vi "Get configuration chain.vi"(8 "error in (no error)":errorcluster, 11 "ServiceManager in":refnum<class "ServiceManager.lvclass">) -> (0 "error out":errorcluster, 1 "class name":string[](array[string]), 2 "configuration chain":variant[](array[variant]), 3 "ServiceManager out":refnum<class "ServiceManager.lvclass">)   [LabVIEW 2012, in "ServiceManager.lvclass"]
doc: "Returns an array of variants containing the configuration clusters of each class in the inheritance chain (lowest child class first), together with an array of all class names in the inheritance chain.\n\nFor classes without configuration cluster, the configuration chain contains empty variants."
uses:
  ServiceManager.lvclass
  Murmex/LabVIEW/Murmex/Murmex/Murmex.lvclass
  ServiceManager.lvclass/ServiceManager.ctl
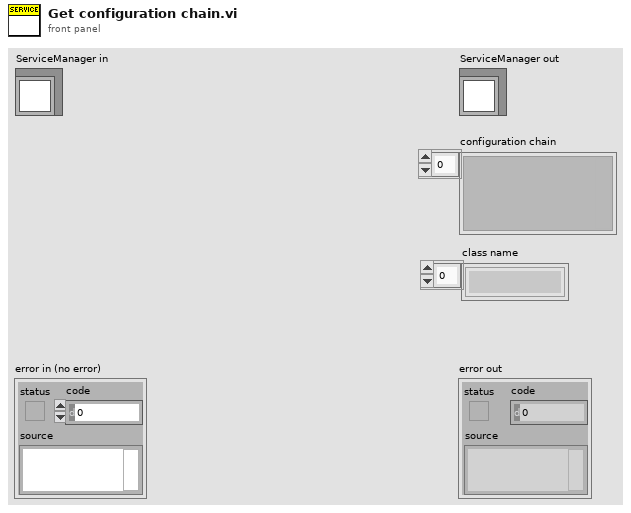
[diagram p1: front panel]
types:
  T1 = typedef "ServiceManager.lvclass/configuration_cluster.ctl" = cluster{"search paths":string[]}
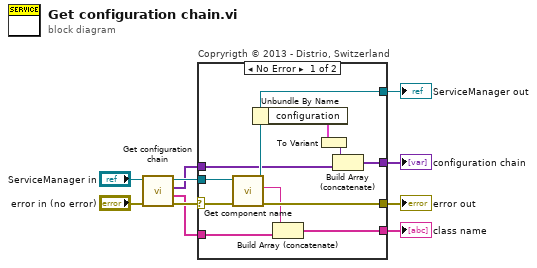
[diagram p0: block diagram]
diagram:
  n1 = call-parent "Get configuration chain.vi"("error in (no error)"="error in (no error)", "MurmexBase in"="ServiceManager in") -> ("error out"=w8:errorcluster, "class name"=w4:string[], "configuration chain"=w5:variant[], "MurmexBase out"=w7:refnum<class "ServiceManager.lvclass">)  [unwired: 6 in]
  n2 = case "Copryrigth © 2013 - Distrio, Switzerland" shown="No Error" w8 {
    selector: w8 -> [w18 w23]
    tunnel: [w17 w23] -> w1
    tunnel: [w15 w22] -> w2
    tunnel: w7 -> [w16 w22]
    tunnel: [w19 _] -> w6
    tunnel: [w13 _] -> w3
    tunnel: w5 -> [w12 _]
    tunnel: w4 -> [w11 _]
    frame No Error {
      n3 = call "Get component name.vi"("error in (no error)"=w18, "Murmex in"=w16) -> ("error out"=w17:errorcluster, "component name"=w14:string, "Murmex out"=w15:refnum<class "ServiceManager.lvclass">)  [unwired: 7 in]
      n4 = Unbundle By Name(w15) -> ("configuration"=w21:T1)
      n5 = Build Array (concatenate)(w14, w11) -> (w13:string[])
      n6 = To Variant(anything=w21) -> (Variant=w20:variant)
      n7 = Build Array (concatenate)(w20, w12) -> (w19:variant[])
    }
    frame Error {
    }
  }
  "error out" <- w1
  "ServiceManager out" <- w2
  "configuration chain" <- w6
  "class name" <- w3
